vi "set reset.vi"(10 "reset":bool, 11 "set":bool) -> (3 "Boolean":bool)   [LabVIEW 2019]
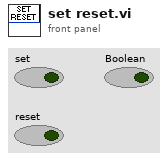
[diagram p1: front panel]
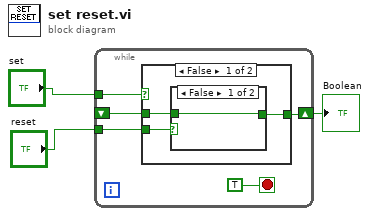
[diagram p0: block diagram]
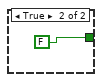
[diagram p2: hidden frame]
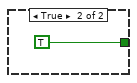
[diagram p3: hidden frame]
diagram:
  n1 = while {
    shift-right: [w6] -> w3
    shift-left: _ -> [w5]
    tunnel: "set" -> [w7]
    tunnel: "reset" -> [w4]
    stop <- TRUE stop-if-true
    n2 = case shown="False" w7 {
      tunnel: [w10 TRUE] -> w6
      tunnel: w5 -> [w9 _]
      tunnel: w4 -> [w11 _]
      frame False {
        n3 = case shown="False" w11 {
          tunnel: [w12 FALSE] -> w10
          tunnel: w9 -> [w12 _]
          frame False {
          }
          frame True {
          }
        }
      }
      frame True {
      }
    }
  }
  "Boolean" <- w3
